vi "Advance past Array.vi"(7 "JSON":string, 9 "Offset":i32) -> (1 "Offset past Array":i32, 3 "State":T1, 6 "Array Start":i32)   [LabVIEW 2015, in "JSONtext.lvlib"]
uses:
  JSONtext.lvlib
  Parsing State.ctl
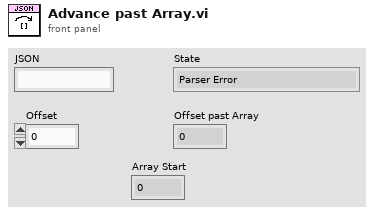
[diagram p1: front panel]
types:
  T1 = typedef "JSONtext.lvlib/Parsing State.ctl" = enum16{"Parser Error", "Object", "Array", "String", "Number/Other", "Leading Whitespace", "Object end", "Array end", "Value end"}
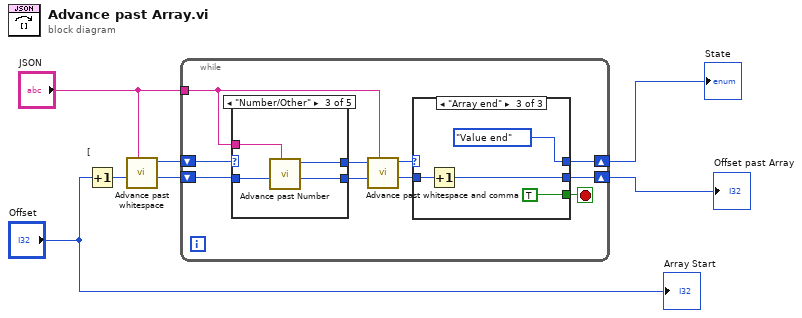
[diagram p0: block diagram]
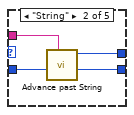
[diagram p3: hidden frame]
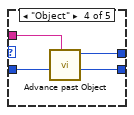
[diagram p4: hidden frame]
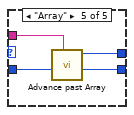
[diagram p5: hidden frame]
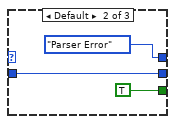
[diagram p7: hidden frame]
diagram:
  n1 = Increment "["(x="Offset") -> (x+1=w3:i32)
  n2 = call "Advance past whitespace.vi"("JSON"="JSON", "Offset"=w3) -> ("Offset of first non-whitespace"=w2:i32, "Parser State"=w4:T1)  [unwired: 8 in]
  n3 = while {
    tunnel: "JSON" -> [w10]
    shift-right: [w15] -> w7
    shift-left: w2 -> [w8]
    shift-right: [w11] -> w5
    shift-left: w4 -> [w9]
    stop <- w14 stop-if-true
    n4 = case shown="\"Number/Other\"" w9 {
      selector: w9 -> [w19 _ _ _ _]
      tunnel: w8 -> [w18 w21 w25 w31 w35]
      tunnel: [w19 w23 w27 w30 w33] -> w13
      tunnel: [w18 w22 w26 w29 w34] -> w12
      tunnel: w10 -> [_ w20 w24 w28 w32]
      frame Default {
      }
      frame "String" {
        n5 = call "Advance past String.vi"("JSON"=w20, "Offset"=w21) -> ("Offset past match"=w22:i32, "State"=w23:T1)  [unwired: 7 in, 1 out]
      }
      frame "Number/Other" {
        n6 = call "Advance past Number.vi"("JSON"=w24, "Offset (0)"=w25) -> ("Offset past match"=w26:i32, "Parser State"=w27:T1)  [unwired: 7 in, 1 out]
      }
      frame "Object" {
        n7 = call "Advance past Object.vi"("JSON"=w28, "Offset"=w31) -> ("Offset past Object"=w29:i32, "State"=w30:T1)  [unwired: 7 in, 1 out]
      }
      frame "Array" {
        n8 = call "Advance past Array.vi"("JSON"=w32, "Offset"=w35) -> ("Offset past Array"=w34:i32, "State"=w33:T1)  [unwired: 7 in, 1 out]
      }
    }
    n9 = call "Advance past whitespace and comma.vi"("JSON"=w10, "Offset"=w12, "State in"=w13) -> ("Offset past match"=w17:i32, "State"=w16:T1)  [unwired: 7 in]
    n10 = case shown="\"Array end\"" w16 {
      selector: w16 -> [w36 _ _]
      tunnel: [_ TRUE TRUE] -> w14
      tunnel: w17 -> [w37 w39 w43]
      tunnel: [w37 w39 w42] -> w15
      tunnel: [w36 Parsing_State."Parser Error" Parsing_State."Value end"] -> w11
      frame "Object".."Number/Other" {
      }
      frame Default {
      }
      frame "Array end" {
        n11 = Increment(x=w43) -> (x+1=w42:i32)
      }
    }
  }
  "State" <- w5
  "Offset past Array" <- w7
  "Array Start" <- "Offset"
